vi "Read ClkDest.vi"(8 "error in (no error)":errorcluster, 11 "NiPxi6682 in":refnum<class "NiPxi6682.lvclass">) -> (0 "error out":errorcluster, 2 "ClkDest":T1={"Term_1"="PXI_Star4", "Term_2"="PXI_Trig0"}, 3 "NiPxi6682 out":refnum<class "NiPxi6682.lvclass">)   [LabVIEW 2014, in "SyncPlugins.lvlib" / "NiPxi6682.lvclass"]
uses:
  NiPxi6682.lvclass
  Typedefs/clClkDest.ctl
  NiPxi6682.lvclass/NiPxi6682.ctl
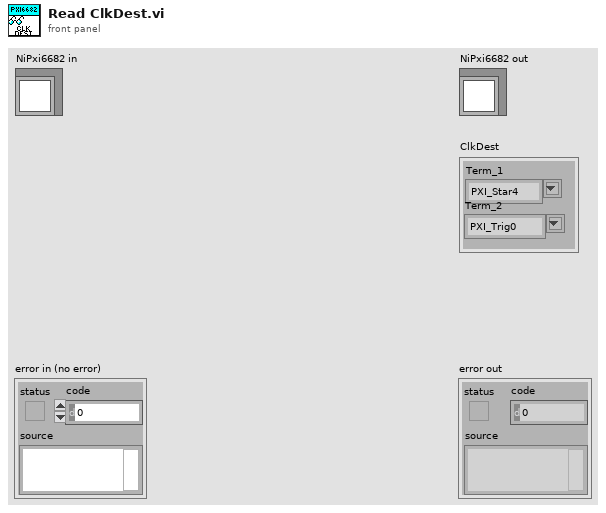
[diagram p1: front panel]
types:
  T1 = typedef "SyncPlugins.lvlib/NiPxi6682.lvclass/clClkDest.ctl" = cluster{"Term_1":string, "Term_2":string}
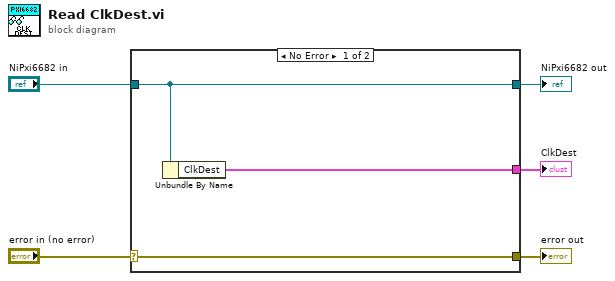
[diagram p0: block diagram]
diagram:
  n1 = case shown="No Error" "error in (no error)" {
    selector: "error in (no error)" -> [w8 w9]
    tunnel: [w8 w9] -> w4
    tunnel: [w7 w10] -> w2
    tunnel: "NiPxi6682 in" -> [w7 w10]
    tunnel: [w6 _] -> w1
    frame No Error {
      n2 = Unbundle By Name(w7) -> ("ClkDest"=w6:T1)
    }
    frame Error {
    }
  }
  "error out" <- w4
  "NiPxi6682 out" <- w2
  "ClkDest" <- w1
